vi "Torque setpoint generation.vi"() -> ()   [LabVIEW 2019]
panel:
  out "D3":dbl
  out "J_equivalent":dbl
  out "D2":dbl
  out "D1":dbl
  in  "GR_diff":dbl
  in  "GR_trans":dbl
  out "C3":dbl
  out "C2":dbl
  in  "slope(degrees)":dbl
  in  "rolling resistance coefficient C_rf":dbl
  in  "gravitational accelaration(m/s^2)":dbl
  in  "mass(kg)":dbl
  out "C1":dbl
  in  "Frontal Area(m^2)":dbl
  in  "density_air(kg/m^3)":dbl
  in  "C_d":dbl
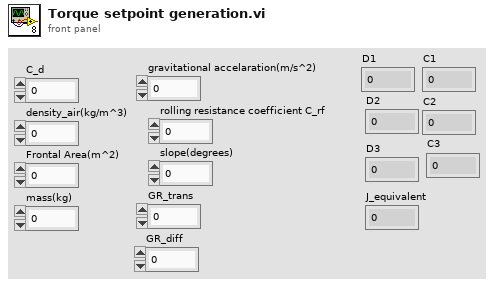
[diagram p1: front panel]
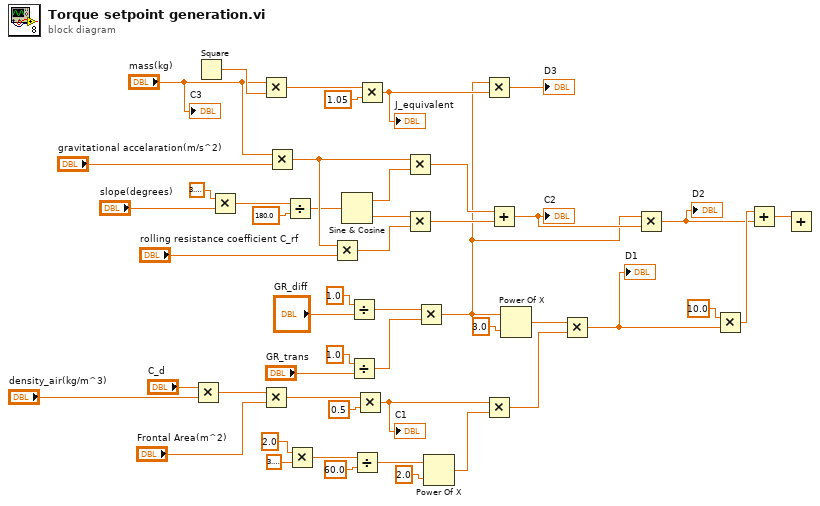
[diagram p0: block diagram]
diagram:
  n1 = Multiply(x="C_d", y="density_air(kg/m^3)") -> (x*y=w47:dbl)
  n2 = Square() -> (x^2=w12:dbl)  [unwired: 1 in]
  n3 = Multiply(x=3.141592653589793, y="slope(degrees)") -> (x*y=w33:dbl)
  n4 = Multiply(x="mass(kg)", y=w12) -> (x*y=w10:dbl)
  n5 = Multiply(x=w47, y="Frontal Area(m^2)") -> (x*y=w45:dbl)
  n6 = Multiply(x="mass(kg)", y="gravitational accelaration(m/s^2)") -> (x*y=w39:dbl)
  n7 = Divide(x=w33, y=180.0 ("x/y")) -> (x/y=w31:dbl)
  n8 = Multiply(x=2.0 ("y"), y=3.141592653589793) -> (x*y=w28:dbl)
  n9 = Multiply(x=w39, y="rolling resistance coefficient C_rf") -> (x*y=w41:dbl)
  n10 = Sine & Cosine(0:w31) -> (1:w38:dbl, 2:w40:dbl)
  n11 = Divide(x=1.0 ("y"), y="GR_diff") -> (x/y=w18:dbl)
  n12 = Divide(x=1.0 ("y"), y="GR_trans") -> (x/y=w17:dbl)
  n13 = Divide(x=w28, y=60.0) -> (x/y=w26:dbl)
  n14 = Multiply(x=w45, y=0.5 ("x*y")) -> (x*y=w24:dbl)
  "C1" <- w24
  n15 = Multiply(x=w10, y=1.05 ("x")) -> (x*y=w8:dbl)
  "J_equivalent" <- w8
  n16 = Multiply(x=w39, y=w38) -> (x*y=w37:dbl)
  n17 = Multiply(x=w40, y=w41) -> (x*y=w36:dbl)
  n18 = Multiply(x=w18, y=w17) -> (x*y=w7:dbl)
  n19 = Power Of X(1:2.0 ("x^y"), 2:w26) -> (0:w23:dbl)
  n20 = Multiply(x=w7, y=w8) -> (x*y=→"D3":dbl)
  n21 = Multiply(x=w24, y=w23) -> (x*y=w14:dbl)
  n22 = Add(x=w37, y=w36) -> (x+y=w13:dbl)
  "C2" <- w13
  n23 = Power Of X(1:3.0 ("x^y"), 2:w7) -> (0:w15:dbl)
  n24 = Multiply(x=w15, y=w14) -> (x*y=w5:dbl)
  "D1" <- w5
  n25 = Multiply(x=w7, y=w13) -> (x*y=w3:dbl)
  "D2" <- w3
  n26 = Multiply(x=10.0, y=w5) -> (x*y=w4:dbl)
  n27 = Add(x=w4, y=w3) -> (x+y=w2:dbl)
  n28 = Add(x=w2) -> ()  [unwired: 1 in, 1 out]
  "C3" <- "mass(kg)"
